vi "createFilenameArray.vi"(0 "No colours":i32, 1 "no x steps":i32, 2 "no z steps":i32, 3 "no y steps":i32, 4 "Base path":path=path "C:/Users/sims01/Desktop/dataAcq") -> (5 "stackFnameArray":path[][][](array[path]), 6 "frameFilenameArray":path[][][][](array[path]), 7 "tifStackFNameArray":path[][][](array[path]))   [LabVIEW 2015]
panel:
  out "size(s)":i32[](array[numeric])
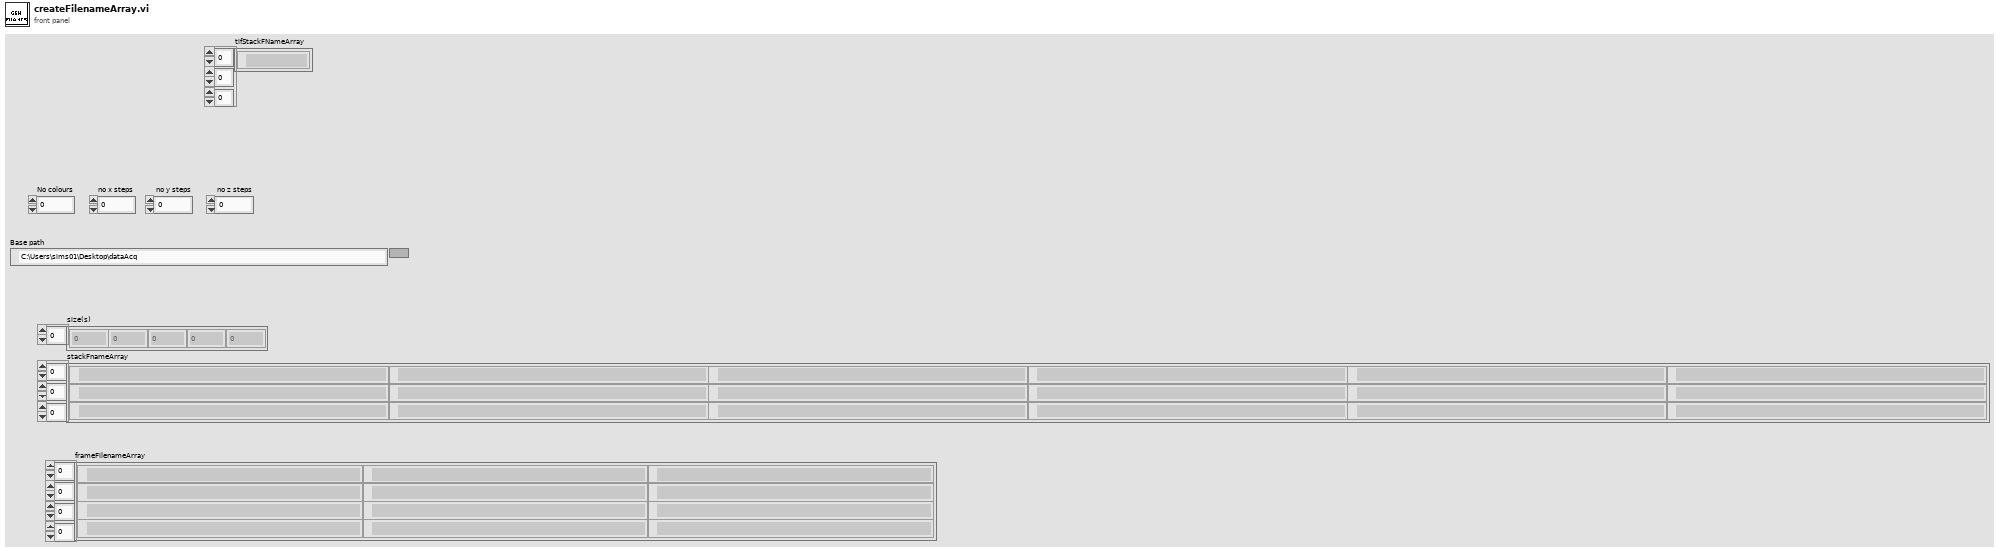
[diagram p1: front panel]
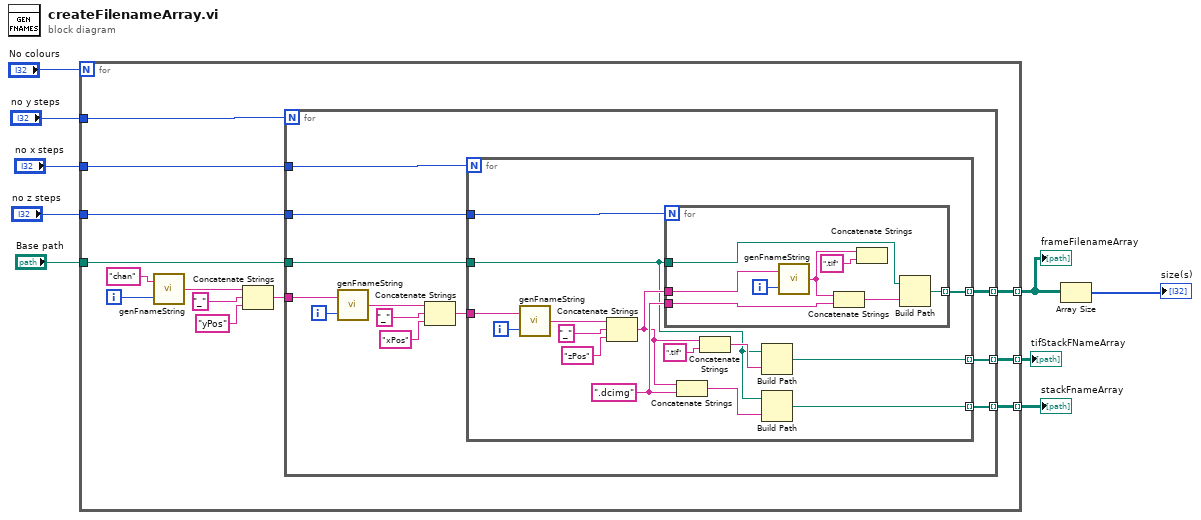
[diagram p0: block diagram]
diagram:
  n1 = for {
    N: "No colours" -> [_]
    tunnel: "no y steps" -> [w22]
    tunnel: "no x steps" -> [w21]
    tunnel: "no z steps" -> [w20]
    tunnel: [w17] -> w5 mode=indexing
    tunnel: "Base path" -> [w16]
    tunnel: [w15] -> w2 mode=indexing
    tunnel: [w14] -> w1 mode=indexing
    i -> [w19]
    n2 = call "genFnameString.vi"("Idx"=w19, "str"="chan") -> ("fName"=w12:string)
    n3 = Concatenate Strings(w12, "_" ("string"), "yPos") -> (w10:string)
    n4 = for {
      N: w22 -> [_]
      tunnel: w21 -> [w34]
      tunnel: w20 -> [w33]
      tunnel: [w31] -> w17 mode=indexing
      tunnel: w16 -> [w30]
      tunnel: [w29] -> w15 mode=indexing
      tunnel: [w28] -> w14 mode=indexing
      tunnel: w10 -> [w27]
      i -> [w32]
      n5 = call "genFnameString.vi"("Idx"=w32, "str"=w27) -> ("fName"=w26:string)
      n6 = Concatenate Strings(w26, "_" ("string"), "xPos") -> (w23:string)
      n7 = for {
        N: w34 -> [_]
        tunnel: w33 -> [w49]
        tunnel: [w47] -> w31 mode=indexing
        tunnel: w30 -> [w36]
        tunnel: [w46] -> w29 mode=indexing
        tunnel: [w35] -> w28 mode=indexing
        tunnel: w23 -> [w45]
        i -> [w48]
        w41 = ".dcimg" ("string")
        n8 = call "genFnameString.vi"("Idx"=w48, "str"=w45) -> ("fName"=w44:string)
        n9 = Concatenate Strings(w44, "_" ("string"), "zPos") -> (w37:string)
        n10 = for {
          N: w49 -> [_]
          tunnel: [w56] -> w47 mode=indexing
          tunnel: w36 -> [w55]
          tunnel: w37 -> [w51]
          tunnel: w41 -> [w50]
          i -> [w57]
          n11 = call "genFnameString.vi"("Idx"=w57, "str"=w51) -> ("fName"=w52:string)
          n12 = Concatenate Strings(w52, w50) -> (w53:string)
          n13 = Concatenate Strings(w52, ".tif" ("string")) -> ()  [unwired: 1 out]
          n14 = Build Path(base path=w55, name or relative path=w53) -> (appended path=w56:path)
        }
        n15 = Concatenate Strings(w37, w41) -> (w40:string)
        n16 = Concatenate Strings(w37, ".tif" ("string")) -> (w38:string)
        n17 = Build Path(base path=w36, name or relative path=w38) -> (appended path=w35:path)
        n18 = Build Path(base path=w36, name or relative path=w40) -> (appended path=w46:path)
      }
    }
  }
  "frameFilenameArray" <- w5
  "stackFnameArray" <- w2
  "tifStackFNameArray" <- w1
  n19 = Array Size(array=w5) -> (size(s)=→"size(s)":i32[])
